vi "Start.vi"(8 "error in (no error)":errorcluster, 11 "Execution in":refnum<data-value>) -> (0 "error out":errorcluster, 3 "Execution out":refnum<data-value>)   [LabVIEW 2015, in "Execution.lvclass"]
uses:
  Execution.lvclass
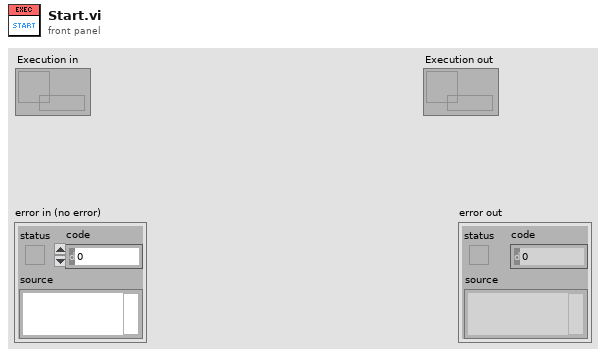
[diagram p1: front panel]
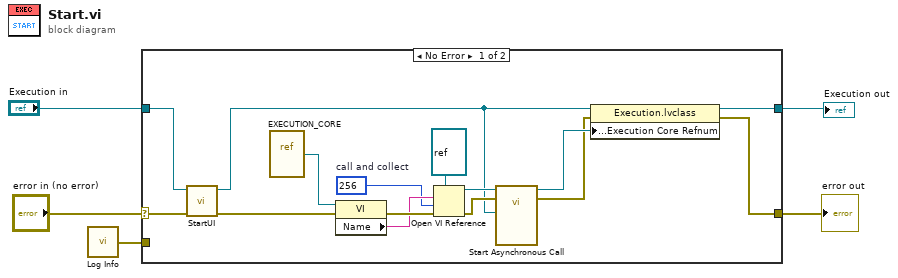
[diagram p0: block diagram]
diagram:
  n1 = call "Log Info.vi"() -> ("error out"=w1:errorcluster)  [unwired: 5 in]
  n2 = case shown="No Error" "error in (no error)" {
    selector: "error in (no error)" -> [w9 w22]
    tunnel: [w10 w22] -> w4
    tunnel: [w12 w21] -> w2
    tunnel: "Execution in" -> [w8 w21]
    tunnel: w1 -> [_ _]
    frame No Error {
      w17 = 256  # call and collect
      n3 = call "StartUI.vi"("error in (no error)"=w9, "Execution in"=w8) -> ("error out"=w6:errorcluster, "Execution out"=w7:refnum<data-value>)  [unwired: 8 in]
      n4 = vi-ref "EXECUTION_CORE.vi"() -> (w18:refnum<vi>)
      n5 = property class="VI"(reference=w18, error in=w6) -> (error out=w20:errorcluster, "Name"=w19:string)  [unwired: 1 out]
      n6 = Open VI Reference(type specifier VI Refnum (for type only)=refnum<vi> refnum ("VI Refnum"), vi path=w19, options=w17, error in (no error)=w20) -> (vi reference=w15:refnum<vi>, error out=w14:errorcluster)  [unwired: 2 in]
      n7 = call-by-ref "Start Asynchronous Call"(reference=w15, error in=w14, "Socket in"=w7) -> (reference out=w13:refnum<vi>, error out=w11:errorcluster)  [unwired: 9 in, 2 out]
      n8 = property class="Execution.lvclass"(reference=w7, error in=w11, "Member Access:Execution Core Refnum"=w13) -> (reference out=w12:refnum<data-value>, error out=w10:errorcluster)
    }
    frame Error {
    }
  }
  "error out" <- w4
  "Execution out" <- w2
